vi "Led On.vi"(8 "error in (no error)":errorcluster, 11 "index":i32) -> (0 "error out":errorcluster, 2 "function_return":i32, 3 "index_out":i32)   [LabVIEW 2013, in "FEMTO_LUCI-10.lvlib"]
doc: "This function switches the LUCI-LED on."
uses:
  FEMTO_LUCI-10.lvlib
  LUCI_10.dll
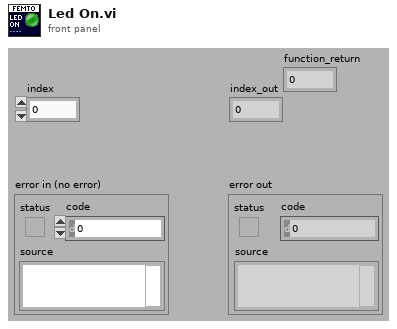
[diagram p1: front panel]
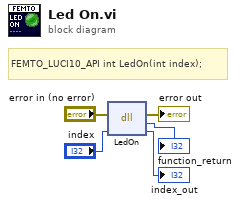
[diagram p0: block diagram]
diagram:
  # "FEMTO_LUCI10_API int LedOn(int index);"
  n1 = dll-call lib="C:/user/patrick/ppms_daq_femto/driver/LUCI_10.*" fn="LedOn"(error in="error in (no error)", "index"="index") -> (error out=→"error out":errorcluster, →"function_return":i32, "index"=→"index_out":i32)  [unwired: 2 in, 1 out]
